vi "invokedotnet.vi"   [LabVIEW 2014]
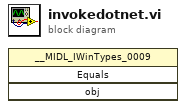
[diagram p0: block diagram]
diagram:
  n1 = invoke class="__MIDL_IWinTypes_0009" method="Equals"() -> ()  [unwired: 4 in, 4 out]
